vi "coaxial_control_4.1.vi"() -> ()   [LabVIEW 2018]
uses:
  <vilib>/DAQmx/read.llb/DAQmx Read (Analog 2D DBL NChan NSamp).vi
  <vilib>/Analysis/NI_AALBase.lvlib
  <vilib>/Analysis/baseanly.llb/Mean (DBL).vi
  <vilib>/Analysis/NI_AALPro.lvlib
  <vilib>/addons/System Identification/NI_SysID.lvlib
  <vilib>/addons/System Identification/Data Preprocess.llb/SI Bandpass Filter (SISO Array).vi
  <vilib>/addons/control/pid/NI_PID_autopid.lvlib
  <vilib>/ptbypt/NI_PtbyPt.lvlib
  <vilib>/DAQmx/create/channels.llb/DAQmx Create Channel (AI-Voltage-Basic).vi
  <vilib>/DAQmx/create/channels.llb/DAQmx Create Channel (CO-Pulse Generation-Frequency).vi
  <vilib>/DAQmx/configure/timing.llb/DAQmx Timing (Sample Clock).vi
  <vilib>/DAQmx/configure/timing.llb/DAQmx Timing (Implicit).vi
  <vilib>/DAQmx/write.llb/DAQmx Write (Counter 1D Frequency NChan 1Samp).vi
panel:
  out "PWM":dbl=0.5
  in  "0 RPM power":dbl=0.01
  in  "0 RPM power":dbl=0.01
  in  "PID gains":T1={"proportional gain (Kc)"=0.002855, "integral time (Ti, min)"=0.003704, "derivative time (Td, min)"=0.000926} {"derivative time (Td, min)" format="%.7f"; "integral time (Ti, min)" format="%.7f"; "proportional gain (Kc)" format="%.7f"}
  in  "output range":cluster{"output high":dbl, "output low":dbl}={"output high"=1158.0, "output low"=1080.0} {"output low" format="%.2f"; "output high" format="%.2f"}
  out "Array":cluster{"[0]":dbl, "[0]":dbl}[](array[cluster])=[{"[0]"=0.5, "[0]"=500.0}, {"[0]"=0.5, "[0]"=500.0}]
  out "?":dbl=0.0036682040382713314 format="%0.4f"
  in  "samples":i32=1000
  in  "rate":dbl=1000.0 format="%0.2f"
  in  "physical channels":tag="Dev1/ai2:1"
  in  "samples per channel":i32=1000
  in  "duty cycle":dbl=0.5 format="%.6f"
  in  "frequency":dbl=500.0 format="%.6f"
  in  "counter":tag="Dev1/ctr1:0"
  in  "stop":bool
  in  "?":i32=1000
  out "RPM 2":dbl
  out "Avg RPM":dbl(graph)=5823.156462005219
  in  "high cutoff RPM":dbl=6500.0 format="%0.3f"
  in  "low cutoff RPM":dbl=5500.0
  in  "setpoint RPM":dbl format="%.2f"
  out "PWM":dbl=0.5
  out "est power peak":dbl=0.004604255842554169 format="%0.4f"
  out "Elapsed Time (s)":dbl=722.9954853057861
  out "Smooth set":dbl
  in  "?":cluster{"output high":dbl, "output low":dbl}={"output high"=1158.0, "output low"=1135.0} {"output low" format="%.2f"; "output high" format="%.2f"}
  in  "?":T1={"proportional gain (Kc)"=0.002855, "integral time (Ti, min)"=0.003704, "derivative time (Td, min)"=0.000926} {"derivative time (Td, min)" format="%.7f"; "integral time (Ti, min)" format="%.7f"; "proportional gain (Kc)" format="%.7f"}
  in  "Phase angle change":dbl format="%.2f"
  in  "Position PID":T1={"proportional gain (Kc)"=0.002855, "integral time (Ti, min)"=0.003704, "derivative time (Td, min)"=0.00926} {"derivative time (Td, min)" format="%.7f"; "integral time (Ti, min)" format="%.7f"; "proportional gain (Kc)" format="%.7f"}
  in  "Position PID bound":cluster{"output high":dbl, "output low":dbl}={"output high"=0.1, "output low"=-0.1} {"output low" min=-0.0001 max=-0.0001 format="%.7f"; "output high" format="%.7f"}
  in  "Speed or pos?":dbl=1.0
  in  "Nominal pwm":dbl=0.557
  in  "sample length":i32=100
  out "RPM":dbl(graph)
  in  "position fineese":dbl=250.0
  in  "Time to subtract":dbl
  out "RPM 3":dbl
  out "RPM  4":dbl(graph)
  out "Avg RPM 2":dbl(graph)=5876.234152924878
  in  "High cut off RPM 2":dbl=6500.0
  in  "Low cut off RPM 2":dbl=5500.0
  # "DAQ PROPERTIES"
  # "ROTOR WITH SPEED AND POSITION CONTROL (LOWER)"
  # "ROTOR WITH SPEED CONTROL (UPPER)"
  # "RPM MEASUREMENT"
  # "RPM MEASUREMENT"
  # "SPEED CONTROLLER"
  # "POSITION CONTROLLER"
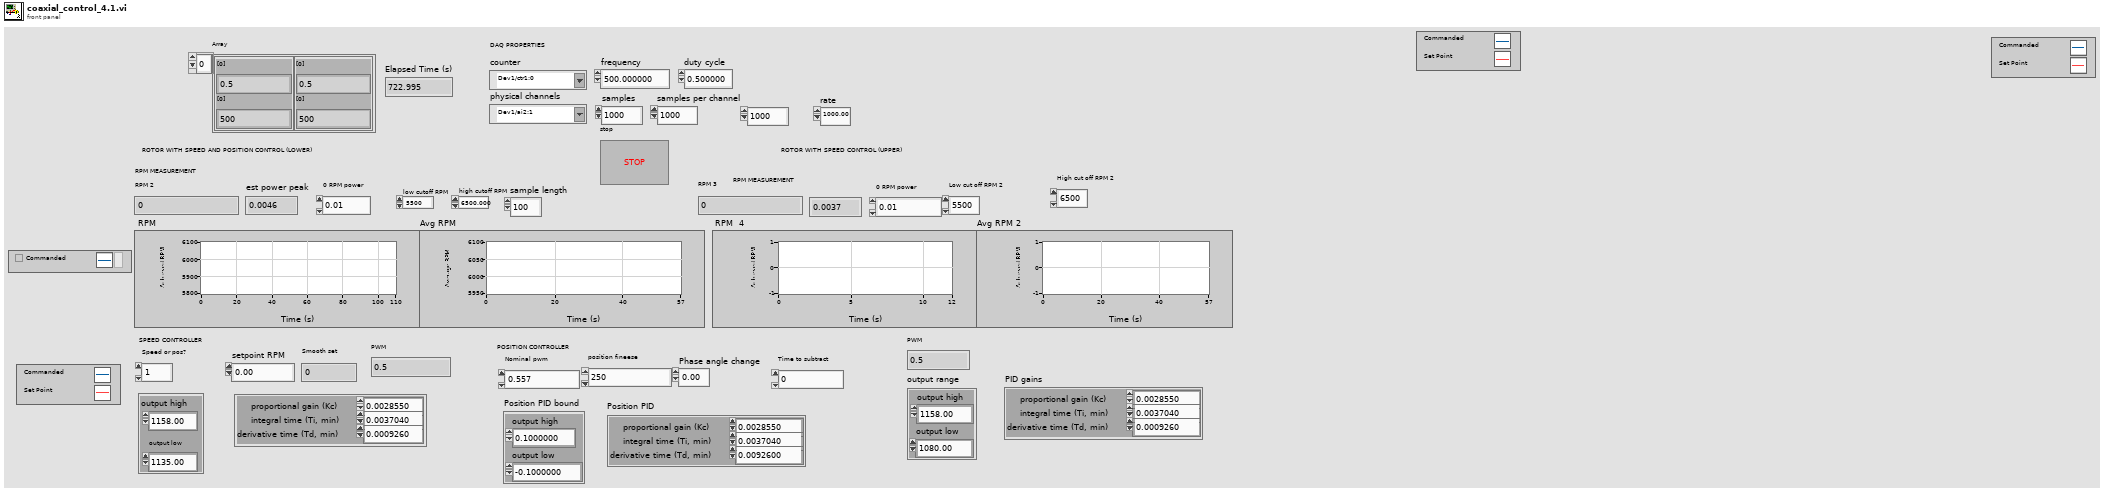
[diagram p1: front panel]
types:
  T1 = cluster{"proportional gain (Kc)":dbl, "integral time (Ti, min)":dbl, "derivative time (Td, min)":dbl}
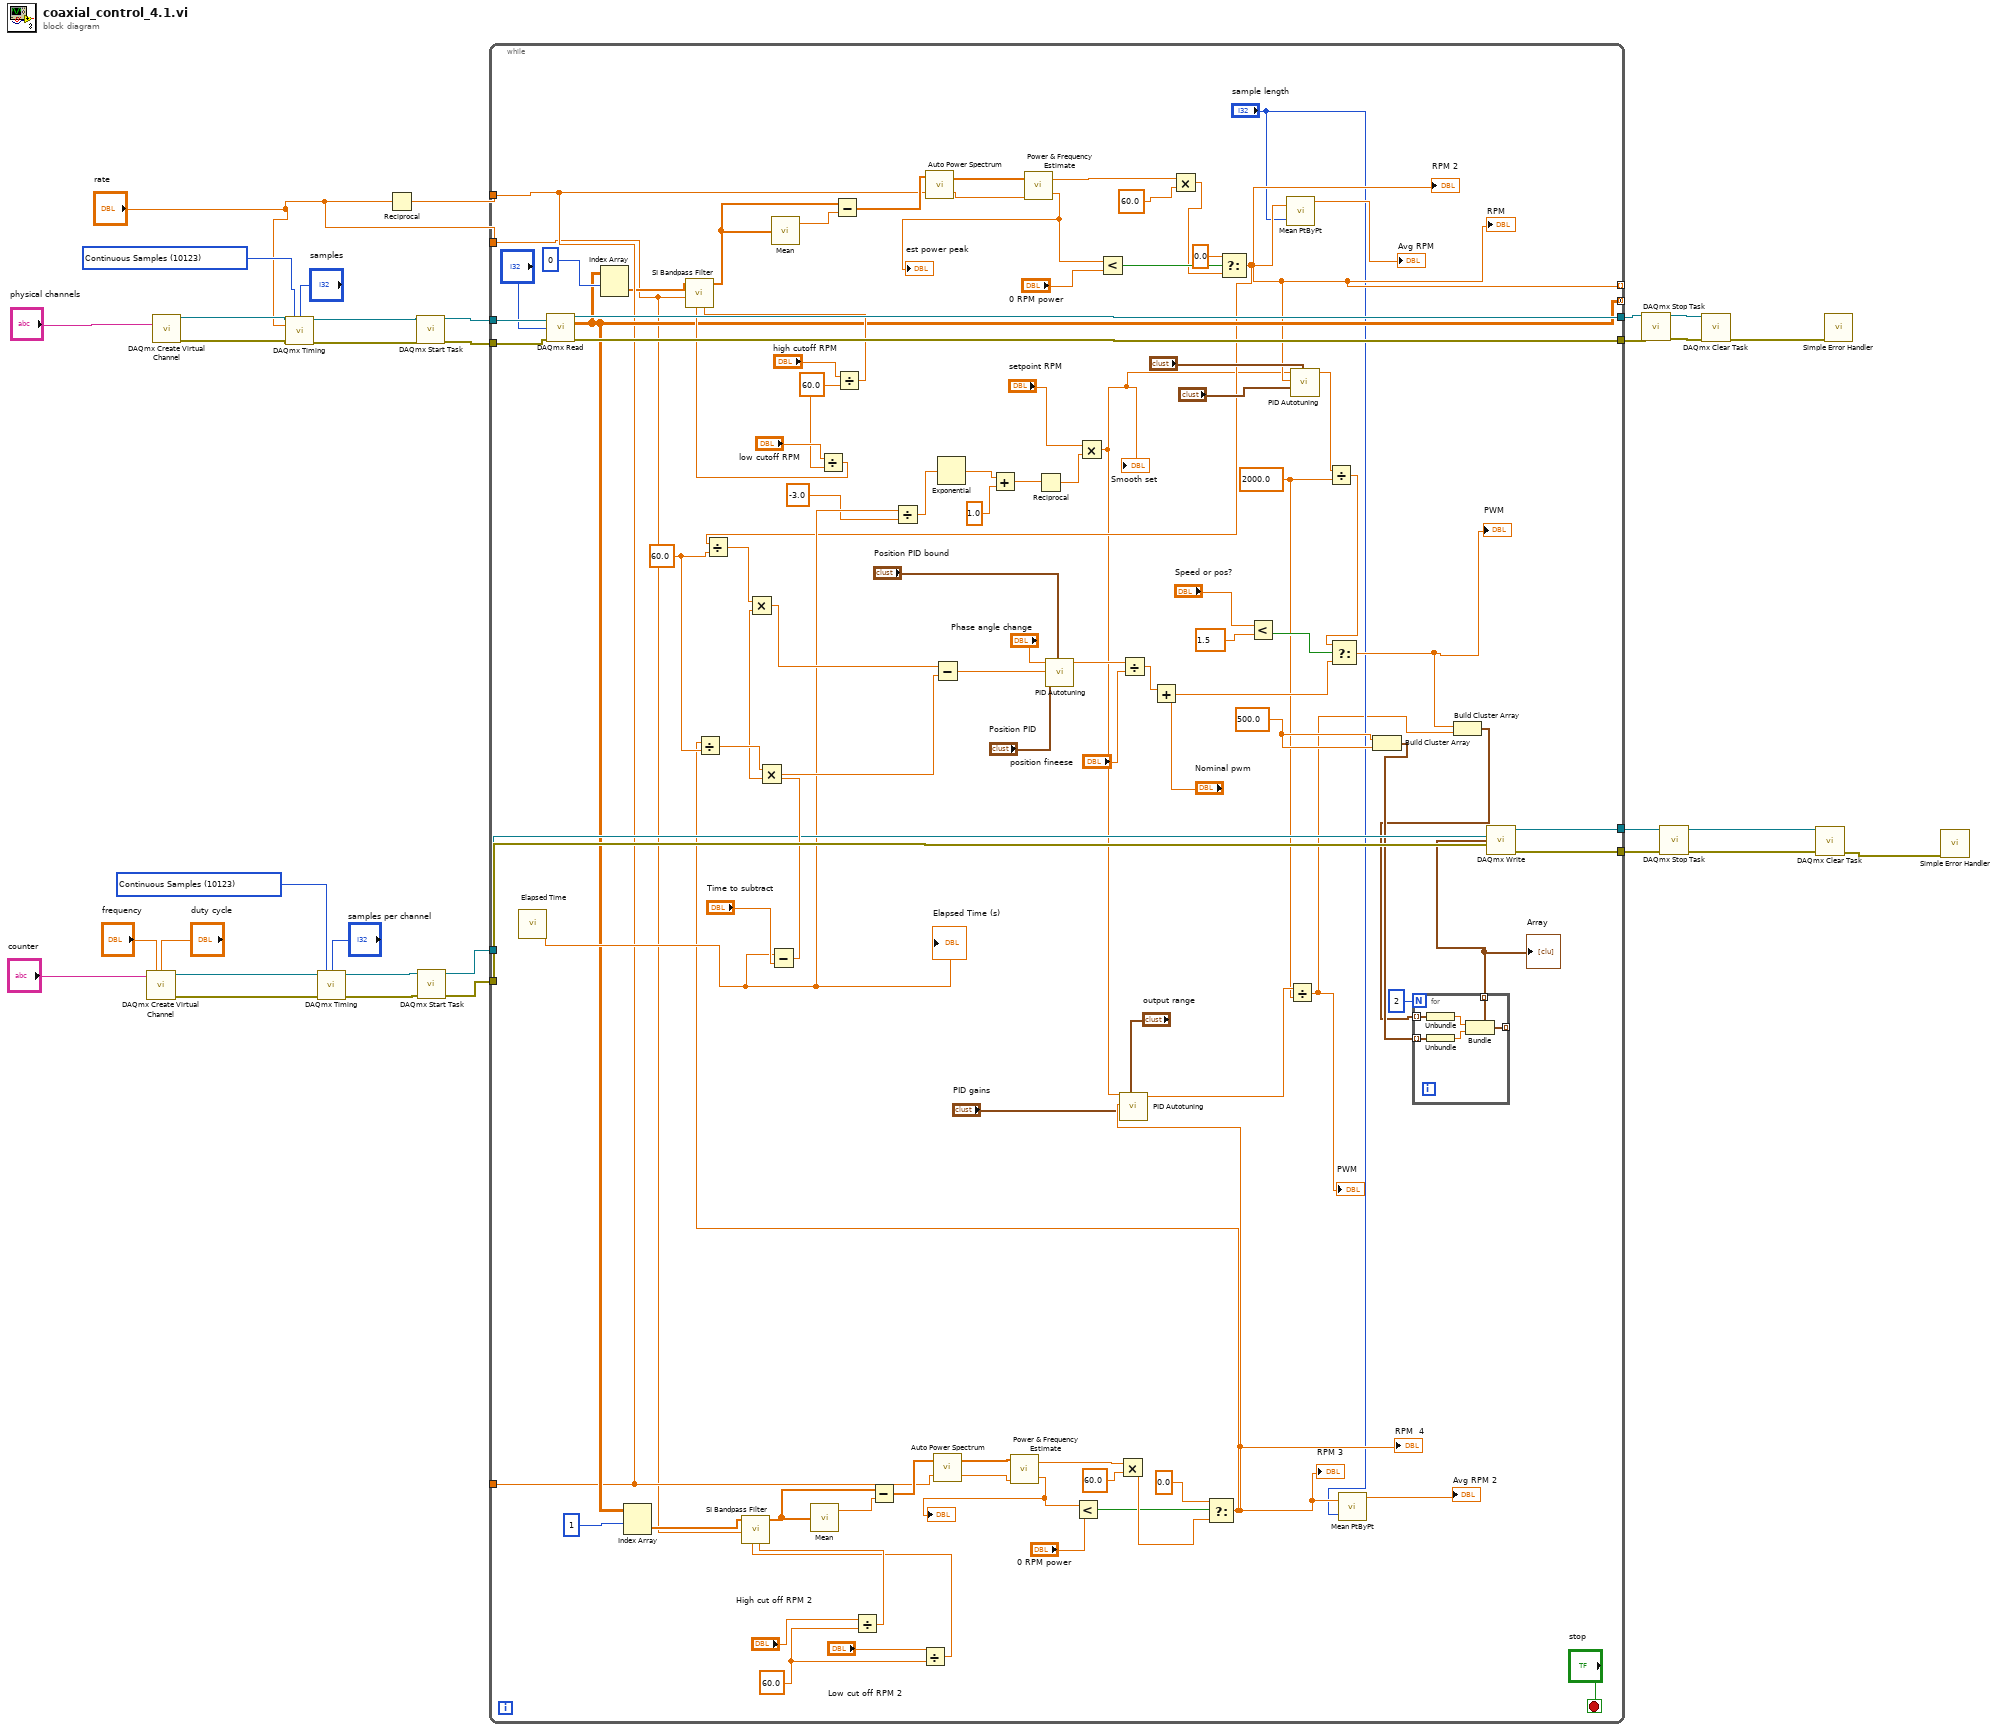
[diagram p0: block diagram]
diagram:
  w5 = 10123 items=["Finite Samples"=10178, "Continuous Samples"=10123, "Hardware Timed Single Point"=12522] ("sample mode")
  w10 = 10123 items=["Finite Samples"=10178, "Continuous Samples"=10123, "Hardware Timed Single Point"=12522] ("sample mode")
  n1 = call-poly <vilib>:"DAQmx Create Virtual Channel.vi"("frequency"="frequency", "duty cycle"="duty cycle", "counter"="counter") -> ("task out"=w32:refnum<k21>, "error out"=w29:errorcluster)  [unwired: 11 in]
  n2 = call-poly <vilib>:"DAQmx Create Virtual Channel.vi"("physical channels"="physical channels") -> ("task out"=w24:refnum<k21>, "error out"=w23:errorcluster)  [unwired: 13 in]
  n3 = call-poly <vilib>:"DAQmx Timing.vi"("task/channels in"=w24, "sample mode"=w5, "samples per channel"="samples", "rate"="rate", "error in"=w23) -> ("task out"=w22:refnum<k21>, "error out"=w21:errorcluster)  [unwired: 9 in]
  n4 = call-poly <vilib>:"DAQmx Timing.vi"("task/channels in"=w32, "sample mode"=w10, "samples per channel"="samples per channel", "error in"=w29) -> ("task out"=w31:refnum<k21>, "error out"=w28:errorcluster)  [unwired: 10 in]
  n5 = Reciprocal(x="rate") -> (1/x=w4:dbl)
  n6 = call <vilib>:"DAQmx Start Task.vi"("task/channels in"=w22, "error in"=w21) -> ("task out"=w20:refnum<k21>, "error out"=w19:errorcluster)  [unwired: 12 in]
  n7 = call <vilib>:"DAQmx Start Task.vi"("task/channels in"=w31, "error in"=w28) -> ("task out"=w30:refnum<k21>, "error out"=w27:errorcluster)  [unwired: 12 in]
  n8 = while {
    tunnel: w30 -> [w78]
    tunnel: w27 -> [w130]
    tunnel: w20 -> [w129]
    tunnel: w19 -> [w128]
    tunnel: [w127] -> w18
    tunnel: [w126] -> w17
    tunnel: w4 -> [w54]
    tunnel: [w56] -> _ mode=concatenating
    tunnel: "rate" -> [w51]
    tunnel: [w43] -> _ mode=indexing
    tunnel: [w77] -> w2
    tunnel: [w76] -> w1
    tunnel: [w54] -> _
    stop <- "stop" stop-if-true
    w46 = 500.0 ("element")
    w62 = 60.0 ("y")
    w82 = 60.0 ("y")
    w88 = 60.0 ("y")
    w37 = 2000.0 ("y")
    n9 = call "Elapsed Time"() -> ("Elapsed Time (s)"=w60:dbl)  [unwired: 12 in, 7 out]
    "Elapsed Time (s)" <- w60
    n10 = call-poly <vilib>:"DAQmx Read.vi"("task/channels in"=w129, "number of samples per channel"="?", "error in"=w128) -> ("task out"=w127:refnum<k21>, "data"=w56:dbl[][], "error out"=w126:errorcluster)  [unwired: 10 in]
    n11 = Index Array(array=w56, index (row)=0) -> (element=w53:dbl[])  [unwired: 1 in]
    n12 = Index Array(array=w56, index (row)=1) -> (element=w52:dbl[])  [unwired: 1 in]
    n13 = Subtract(x=w60, y="Time to subtract") -> (x-y=w79:dbl)
    n14 = Divide(x="low cutoff RPM", y=w82) -> (x/y=w81:dbl)
    n15 = Divide(x="high cutoff RPM", y=w82) -> (x/y=w84:dbl)
    n16 = call-poly <vilib>:"SI Bandpass Filter.vi"("high cutoff freq"=w84, "low cutoff freq"=w81, "sampling rate (Hz)"=w51, "stimulus signal in"=w53) -> ("stimulus signal out"=w120:dbl[])  [unwired: 5 in, 2 out]
    n17 = call-poly <vilib>:"Mean.vi"("X"=w120) -> ("mean"=w124:dbl)  [unwired: 1 out]
    n18 = Subtract(x=w120, y=w124) -> (x-y=w121:dbl[])
    n19 = Divide(x="High cut off RPM 2", y=w62) -> (x/y=w63:dbl)
    n20 = Divide(x=w60, y=-3.0 ("x")) -> (x/y=w113:dbl)
    n21 = Divide(x="Low cut off RPM 2", y=w62) -> (x/y=w61:dbl)
    n22 = call-poly <vilib>:"SI Bandpass Filter.vi"("high cutoff freq"=w63, "low cutoff freq"=w61, "sampling rate (Hz)"=w51, "stimulus signal in"=w52) -> ("stimulus signal out"=w74:dbl[])  [unwired: 5 in, 2 out]
    n23 = call-poly <vilib>:"Mean.vi"("X"=w74) -> ("mean"=w75:dbl)  [unwired: 1 out]
    n24 = Subtract(x=w74, y=w75) -> (x-y=w73:dbl[])
    n25 = call <vilib>:"Auto Power Spectrum.vi"("dt"=w54, "Signal (V)"=w121) -> ("df"=w118:dbl, "Power Spectrum (V^2 rms)"=w123:dbl[])
    n26 = call <vilib>:"Auto Power Spectrum.vi"("dt"=w54, "Signal (V)"=w73) -> ("df"=w71:dbl, "Power Spectrum (V^2 rms)"=w72:dbl[])
    n27 = Exponential(1:w113) -> (0:w111:dbl)
    n28 = Add(x=w111, y=1.0) -> (x+y=w110:dbl)
    n29 = call <vilib>:"Power & Frequency Estimate.vi"("df"=w71, "Power Spectrum (V^2 rms)"=w72) -> ("est power peak"=w50:dbl, "est frequency peak"=w70:dbl)  [unwired: 4 in]
    "?" <- w50
    n30 = call <vilib>:"Power & Frequency Estimate.vi"("df"=w118, "Power Spectrum (V^2 rms)"=w123) -> ("est power peak"=w115:dbl, "est frequency peak"=w119:dbl)  [unwired: 4 in]
    "est power peak" <- w115
    n31 = Reciprocal(x=w110) -> (1/x=w109:dbl)
    n32 = Less?(x=w50, y="0 RPM power") -> (x < y?=w66:bool)
    n33 = Multiply(x="setpoint RPM", y=w109) -> (x*y=w41:dbl)
    "Smooth set" <- w41
    n34 = Less?(x=w115, y="0 RPM power") -> (x < y?=w117:bool)
    n35 = Multiply(x=w70, y=60.0) -> (x*y=w67:dbl)
    n36 = Multiply(x=w119, y=60.0) -> (x*y=w114:dbl)
    n37 = Select(t=0.0, s=w66, f=w67) -> (s? t:f=w42:dbl)
    "RPM 3" <- w42
    "RPM  4" <- w42
    n38 = Divide(x=w42, y=w88) -> (x/y=w86:dbl)
    n39 = Multiply(x=w86, y=w79) -> (x*y=w95:dbl)
    n40 = call <vilib>:"PID Autotuning.vi"("output range"="output range", "PID gains"="PID gains", "process variable"=w42, "setpoint"=w41) -> ("output"=w38:dbl)  [unwired: 4 in, 3 out]
    n41 = Select(t=0.0, s=w117, f=w114) -> (s? t:f=w43:dbl)
    "RPM 2" <- w43
    "RPM" <- w43
    n42 = Divide(x=w43, y=w88) -> (x/y=w89:dbl)
    n43 = Multiply(x=w89, y=w79) -> (x*y=w96:dbl)
    n44 = Subtract(x=w96, y=w95) -> (x-y=w93:dbl)
    n45 = call <vilib>:"PID Autotuning.vi"("output range"="Position PID bound", "PID gains"="Position PID", "process variable"=w93, "setpoint"="Phase angle change") -> ("output"=w91:dbl)  [unwired: 4 in, 3 out]
    n46 = Divide(x=w91, y="position fineese") -> (x/y=w92:dbl)
    n47 = Add(x=w92, y="Nominal pwm") -> (x+y=w99:dbl)
    n48 = Less?(x="Speed or pos?", y=1.5) -> (x < y?=w100:bool)
    n49 = call <vilib>:"Mean PtByPt.vi"("x"=w43, "sample length"="sample length") -> ("mean"=→"Avg RPM":dbl)  [unwired: 2 in, 1 out]
    n50 = Divide(x=w38, y=w37) -> (x/y=w33:dbl)
    "PWM" <- w33
    n51 = call <vilib>:"PID Autotuning.vi"("output range"="?", "PID gains"="?", "process variable"=w43, "setpoint"=w41) -> ("output"=w107:dbl)  [unwired: 4 in, 3 out]
    n52 = Divide(x=w107, y=w37) -> (x/y=w98:dbl)
    n53 = Select(t=w98, s=w100, f=w99) -> (s? t:f=w47:dbl)
    "PWM" <- w47
    n54 = call <vilib>:"Mean PtByPt.vi"("x"=w42, "sample length"="sample length") -> ("mean"=→"Avg RPM 2":dbl)  [unwired: 2 in, 1 out]
    n55 = Build Cluster Array(w46, w46) -> (w45:cluster{"element":dbl}[])
    n56 = Build Cluster Array(w47, w33) -> (w44:cluster{dbl}[])
    n57 = for {
      N: 2 -> [_]
      tunnel: w44 -> [w136] mode=indexing
      tunnel: w45 -> [w135] mode=indexing
      tunnel: [w132] -> _ mode=indexing
      tunnel: [w132] -> w48 mode=indexing
      n58 = Unbundle(w136) -> (w134:dbl)
      n59 = Unbundle(w135) -> ("element"=w133:dbl)
      n60 = Bundle(w134, "element"=w133) -> (w132:cluster{dbl, "element":dbl})  [unwired: 1 out]
    }
    "Array" <- w48
    n61 = call-poly <vilib>:"DAQmx Write.vi"("task/channels in"=w78, "data"=w48, "error in"=w130) -> ("task out"=w77:refnum<k21>, "error out"=w76:errorcluster)  [unwired: 10 in, 1 out]
  }
  n62 = call <vilib>:"DAQmx Stop Task.vi"("task/channels in"=w18, "error in"=w17) -> ("task out"=w16:refnum<k21>, "error out"=w15:errorcluster)  [unwired: 12 in]
  n63 = call <vilib>:"DAQmx Stop Task.vi"("task/channels in"=w2, "error in"=w1) -> ("task out"=w26:refnum<k21>, "error out"=w25:errorcluster)  [unwired: 12 in]
  n64 = call <vilib>:"DAQmx Clear Task.vi"("task in"=w16, "error in"=w15) -> ("error out"=w6:errorcluster)  [unwired: 13 in]
  n65 = call <vilib>:"DAQmx Clear Task.vi"("task in"=w26, "error in"=w25) -> ("error out"=w9:errorcluster)  [unwired: 13 in]
  n66 = call <vilib>:"Simple Error Handler.vi"("error in (no error)"=w6) -> ()  [unwired: 4 in, 5 out]
  n67 = call <vilib>:"Simple Error Handler.vi"("error in (no error)"=w9) -> ()  [unwired: 4 in, 5 out]
